vi "CSC_SetDHvars.vi"(8 "error in (no error)":errorcluster, 10 "KnownDHVars":T3(array[cluster]), 11 "CSC in":refnum<class "CableSerialChain.lvclass">) -> (0 "error out":errorcluster, 3 "CSC out":refnum<class "CableSerialChain.lvclass">)   [LabVIEW 2015, in "CableSerialChain.lvclass"]
uses:
  CableSerialChain.lvclass
  Body/DH_parameters.ctl
  Body/PointOnBody.ctl
  CableSerialChain.lvclass/CableSerialChain.ctl
  Body/Bodies.lvclass
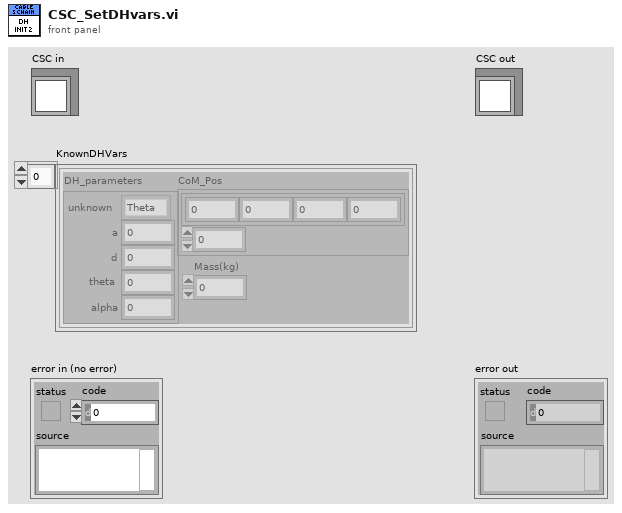
[diagram p1: front panel]
types:
  T1 = typedef "Bodies.lvclass/DH_parameters.ctl" = cluster{"unknown":enum16{"Theta", "Alpha", "a", "d"}, "a":dbl, "d":dbl, "alpha":dbl, "theta":dbl}
  T2 = typedef "Bodies.lvclass/PointOnBody.ctl" = cluster{"Coord4":dbl[], "ID":i32}
  T3 = cluster{"DH_parameters":T1, "CoM_Pos":T2, "Mass(kg)":dbl}[]
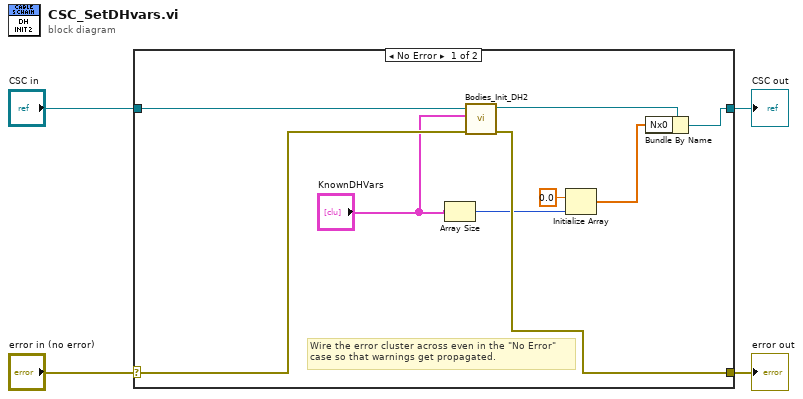
[diagram p0: block diagram]
diagram:
  n1 = case shown="No Error" "error in (no error)" {
    selector: "error in (no error)" -> [w12 w15]
    tunnel: [w11 w15] -> w3
    tunnel: [w13 w14] -> w1
    tunnel: "CSC in" -> [w6 w14]
    frame No Error {
      # "Wire the error cluster across even in the \"No Error\"\ncase so that warnings get propagated."
      n2 = Array Size(array="KnownDHVars") -> (size(s)=w10:i32)
      n3 = call "Bodies_Init_DH2.vi"("error in (no error)"=w12, "KnownDHVars"="KnownDHVars", "Body.lvclass In"=w6) -> ("error out"=w11:errorcluster, "Body.lvclass Out"=w5:refnum<class "CableSerialChain.lvclass">)  [unwired: 7 in]
      n4 = Initialize Array(0.0 ("element"), w10) -> (w8:dbl[])
      n5 = Bundle By Name(cluster=w5, "Nx0"=w8) -> (w13:refnum<class "CableSerialChain.lvclass">)
    }
    frame Error {
    }
  }
  "error out" <- w3
  "CSC out" <- w1
